vi "QMgr_Construct.vi"() -> (3 "queue out":refnum<queue>)   [LabVIEW 2012, in "MB Master.lvlib" / "MB_Master_TCP.lvclass"]
uses:
  MB_Master_TCP.lvclass
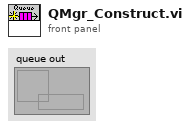
[diagram p1: front panel]
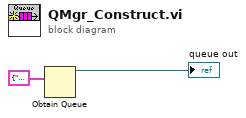
[diagram p0: block diagram]
diagram:
  n1 = Obtain Queue(element data type=cluster{"cmd":string, "data":variant} {"cmd"="", "data"=variant}) -> (queue out=→"queue out":refnum<queue>)  [unwired: 4 in, 2 out]
